vi "DistanceDataAcquisition.vi"(8 "Echo Term":tag="Dev1/ctr1", 11 "Trigger Term":tag="Dev1/ctr0") -> (4 "Distance (IN)":dbl)   [LabVIEW 2014]
uses:
  <vilib>/DAQmx/create/channels.llb/DAQmx Create Channel (CO-Pulse Generation-Time).vi
  <vilib>/DAQmx/configure/timing.llb/DAQmx Timing (Implicit).vi
  <vilib>/DAQmx/create/channels.llb/DAQmx Create Channel (CI-Pulse Width).vi
  <vilib>/DAQmx/read.llb/DAQmx Read (Counter DBL 1Chan 1Samp).vi
panel:
  out "Distance Visual":dbl(slide) scale=0.0..25.0
  # "Connect to the OUT terminal of this counter"
  # "Connect to the GATE terminal of this counter"
  # "The ultrasonic sensor used in this program is the 4 terminal HC-SR04 model.\nThis allows easy connections to dedicated counter input and counter output\nterminals.  It is also necessary to provide +5V and ground."
  # "Image:\nhttp://www.ecrater.com/p/11851880/arduino-ultrasonic-module-hc-sr04"
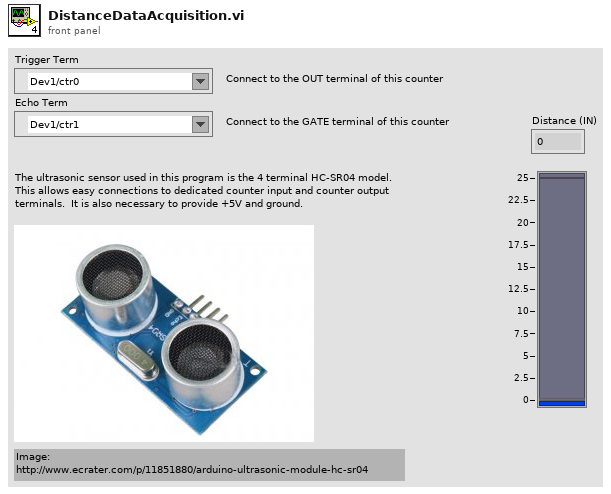
[diagram p1: front panel]
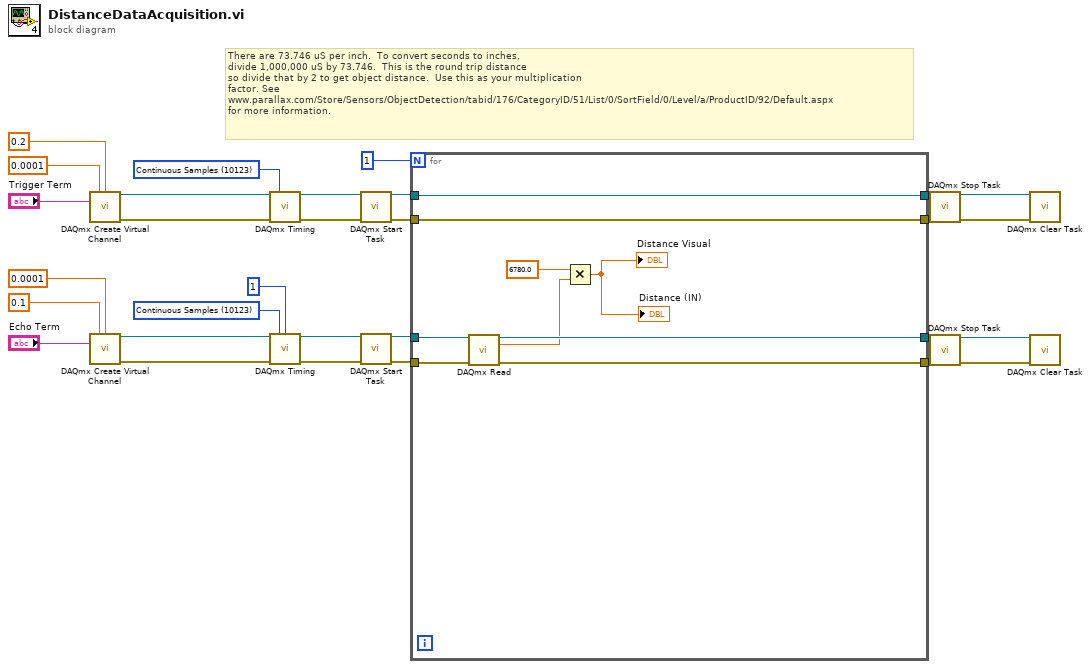
[diagram p0: block diagram]
diagram:
  w11 = 10123 items=["Finite Samples"=10178, "Continuous Samples"=10123, "Hardware Timed Single Point"=12522] ("sample mode")
  w25 = 10123 items=["Finite Samples"=10178, "Continuous Samples"=10123, "Hardware Timed Single Point"=12522] ("sample mode")
  # "There are 73.746 uS per inch.  To convert seconds to inches,\ndivide 1,000,000 uS by 73.746.  This is the round trip distance\nso divide that by 2 to get object distance.  Use this as your multiplication\nfactor. See \nwww.parallax.com/Store/Sensors/ObjectDetection/tabid/176/CategoryID/51/List/0/SortField/0/Level/a/ProductID/92/Default.aspx\nfor more information."
  n1 = call-poly <vilib>:"DAQmx Create Virtual Channel.vi"("high time"=0.0001, "low time"=0.2, "counter"="Trigger Term") -> ("task out"=w26:refnum<k21>, "error out"=w27:errorcluster)  [unwired: 11 in]
  n2 = call-poly <vilib>:"DAQmx Create Virtual Channel.vi"("maximum value"=0.1, "minimum value"=0.0001, "counter"="Echo Term") -> ("task out"=w12:refnum<k21>, "error out"=w13:errorcluster)  [unwired: 11 in]
  n3 = call-poly <vilib>:"DAQmx Timing.vi"("task/channels in"=w26, "sample mode"=w25, "error in"=w27) -> ("task out"=w23:refnum<k21>, "error out"=w24:errorcluster)  [unwired: 11 in]
  n4 = call-poly <vilib>:"DAQmx Timing.vi"("task/channels in"=w12, "sample mode"=w11, "samples per channel"=1, "error in"=w13) -> ("task out"=w9:refnum<k21>, "error out"=w10:errorcluster)  [unwired: 10 in]
  n5 = call <vilib>:"DAQmx Start Task.vi"("task/channels in"=w23, "error in"=w24) -> ("task out"=w15:refnum<k21>, "error out"=w3:errorcluster)  [unwired: 12 in]
  n6 = call <vilib>:"DAQmx Start Task.vi"("task/channels in"=w9, "error in"=w10) -> ("task out"=w17:refnum<k21>, "error out"=w20:errorcluster)  [unwired: 12 in]
  n7 = for {
    N: 1 -> [_]
    tunnel: w20 -> [w39]
    tunnel: [w36] -> w19
    tunnel: [w38] -> w18
    tunnel: w17 -> [w37]
    tunnel: [w35] -> w16
    tunnel: w15 -> [w35]
    tunnel: w3 -> [w34]
    tunnel: [w34] -> w2
    n8 = call-poly <vilib>:"DAQmx Read.vi"("task/channels in"=w37, "error in"=w39) -> ("task out"=w38:refnum<k21>, "data"=w32:dbl, "error out"=w36:errorcluster)  [unwired: 11 in]
    n9 = Multiply(x=6780.0 ("y"), y=w32) -> (x*y=→"Distance Visual" →"Distance (IN)":dbl)
  }
  n10 = call <vilib>:"DAQmx Stop Task.vi"("task/channels in"=w16, "error in"=w2) -> ("task out"=w22:refnum<k21>, "error out"=w21:errorcluster)  [unwired: 12 in]
  n11 = call <vilib>:"DAQmx Stop Task.vi"("task/channels in"=w18, "error in"=w19) -> ("task out"=w5:refnum<k21>, "error out"=w4:errorcluster)  [unwired: 12 in]
  n12 = call <vilib>:"DAQmx Clear Task.vi"("task in"=w22, "error in"=w21) -> ()  [unwired: 13 in, 1 out]
  n13 = call <vilib>:"DAQmx Clear Task.vi"("task in"=w5, "error in"=w4) -> ()  [unwired: 13 in, 1 out]
